vi "Counter.Settings.vi"(6 "Action":enum8{"Get", "Set"}(ring), 8 "error in":errorcluster, 10 "Max Count":dbl, 11 "Parent Ref":T1=18446744073709551615 format="%.0x") -> (0 "error out":errorcluster, 2 "Max Count":dbl, 3 "Parent Ref Out":T1=18446744073709551615 format="%.0x")   [LabVIEW 2015, in "Protection and Counter Support System Explorer.lvlib"]
uses:
  Protection and Counter Support System Explorer.lvlib
  <vilib>/NI Veristand/Custom Device API/Custom Device Item Ref.ctl
  Shared/Properties Lookup.vi
  <vilib>/NI Veristand/Custom Device API/Get Item Property (Double).vi
  <vilib>/NI Veristand/Custom Device API/Set Item Property (Double).vi
  <vilib>/NI VeriStand/Custom Device API/Custom Device API.lvlib
  Shared/Protection and Counter Support Shared.lvlib
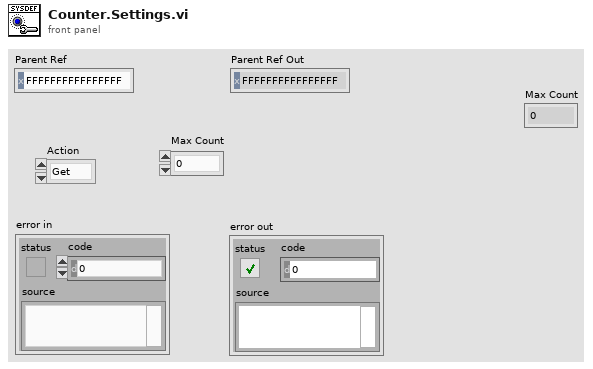
[diagram p1: front panel]
types:
  T1 = typedef "Custom Device API.lvlib/Custom Device Item Ref.ctl" = u64
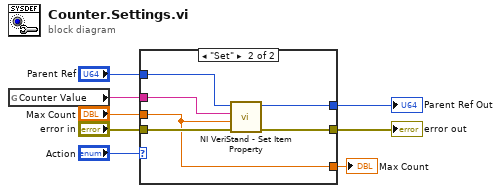
[diagram p0: block diagram]
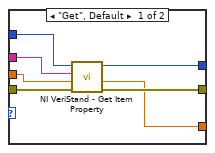
[diagram p2: hidden frame]
diagram:
  n1 = global read "Properties Lookup.vi" "Counter Value"() -> (w4:string)
  n2 = case shown="\"Set\"" "Action" {
    tunnel: "error in" -> [w15 w21]
    tunnel: [w10 w20] -> w7
    tunnel: [w11 w19] -> w6
    tunnel: "Parent Ref" -> [w12 w18]
    tunnel: w4 -> [w13 w17]
    tunnel: "Max Count" -> [w14 w16]
    tunnel: [w9 w16] -> w1
    frame "Get", Default {
      n3 = call-poly <vilib>:"NI VeriStand - Get Item Property.vi"("error in (no error)"=w15, "Default Value"=w14, "Property Name"=w13, "Item Ref in"=w12) -> ("error out"=w10:errorcluster, "Value"=w9:dbl, "Item Ref out"=w11:T1)  [unwired: 4 in, 1 out]
    }
    frame "Set" {
      n4 = call-poly <vilib>:"NI VeriStand - Set Item Property.vi"("error in (no error)"=w21, "Value"=w16, "Property Name"=w17, "Item Ref in"=w18) -> ("error out"=w20:errorcluster, "Item Ref out"=w19:T1)  [unwired: 5 in, 1 out]
    }
  }
  "error out" <- w7
  "Parent Ref Out" <- w6
  "Max Count" <- w1
